vi "Convert Trajectory Data 4.0.vi"(1 "pre 4.0":T3(array[cluster])) -> (0 "post 4.0":T1)   [LabVIEW 2025]
uses:
  Types/Segment Type.ctl
  Types/Trajectory Data.ctl
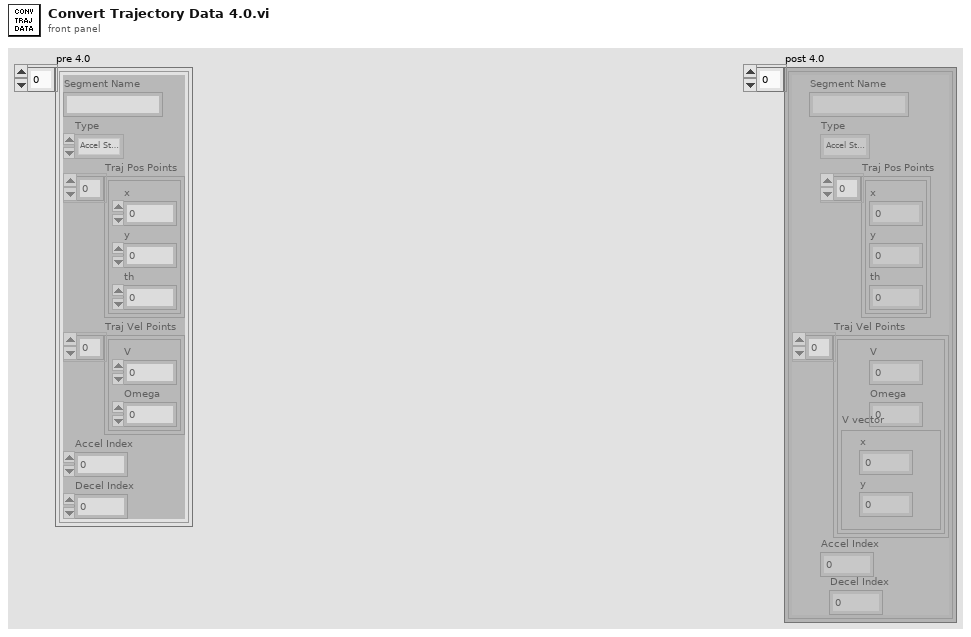
[diagram p1: front panel]
types:
  T1 = typedef "Trajectory Data.ctl" = cluster{"Segment Name":string, "Type":T2, "Traj Pos Points":cluster{"x":dbl, "y":dbl, "th":dbl}[], "Traj Vel Points":cluster{"V":dbl, "Omega":dbl, "V vector":cluster{"y":dbl, "x":dbl}}[], "Accel Index":i32, "Decel Index":i32}[]
  T2 = typedef "Segment Type.ctl" = enum16{"Accel Straight", "Const Straight", "Blend", "Circle", "Bezier"}
  T3 = cluster{"Segment Name":string, "Type":T2, "Traj Pos Points":cluster{"x":dbl, "y":dbl, "th":dbl}[], "Traj Vel Points":cluster{"V":dbl, "Omega":dbl}[], "Accel Index":i32, "Decel Index":i32}[]
  T4 = cluster{"Segment Name":string, "Type":T2, "Traj Pos Points":cluster{"x":dbl, "y":dbl, "th":dbl}[], "Traj Vel Points":cluster{"V":dbl, "Omega":dbl, "V vector":cluster{"y":dbl, "x":dbl}}[], "Accel Index":i32, "Decel Index":i32}
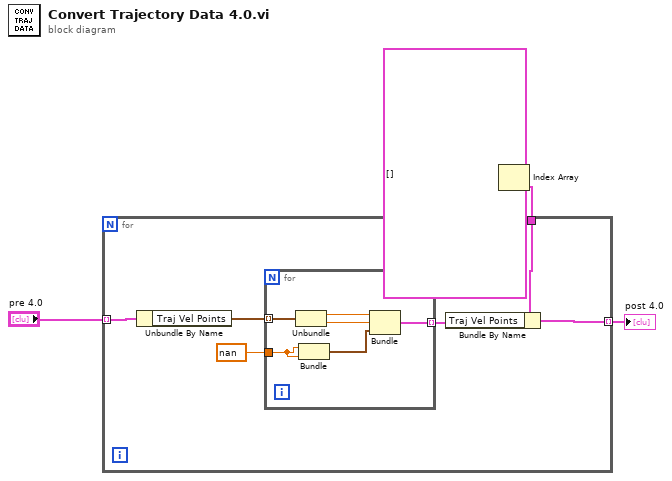
[diagram p0: block diagram]
diagram:
  n1 = Index Array(array=T1 [] ("post 4.0")) -> (element=w2:T4)  [unwired: 1 in]
  n2 = for {
    tunnel: "pre 4.0" -> [w10] mode=indexing
    tunnel: w2 -> [w9]
    tunnel: [w5] -> w1 mode=indexing
    n3 = Unbundle By Name(w10) -> ("Traj Vel Points"=w8:cluster{"V":dbl, "Omega":dbl}[])
    n4 = for {
      tunnel: w8 -> [w16] mode=indexing
      tunnel: nan -> [w15]
      tunnel: [w11] -> w6 mode=indexing
      n5 = Unbundle(w16) -> ("V"=w14:dbl, "Omega"=w13:dbl)
      n6 = Bundle(w15, w15) -> (w12:cluster{dbl, dbl})  [unwired: 1 in]
      n7 = Bundle("V"=w14, "Omega"=w13, w12) -> (w11:cluster{"V":dbl, "Omega":dbl, cluster{dbl, dbl}})  [unwired: 1 in]
    }
    n8 = Bundle By Name(cluster=w9, "Traj Vel Points"=w6) -> (w5:T4)
  }
  "post 4.0" <- w1
